vi "charsquential.vi"() -> ()   [LabVIEW 2012]
uses:
  <vilib>/addons/Modulation/Digital/General/MT Generate PSK System Parameters(M).vi
  <instrlib>/niUSRP/niUSRP Write Tx Data (CDB Cluster).vi
  <vilib>/addons/Modulation/niDMT.lvlib
panel:
  out "Enter control signal (1,2 or 3)\n1. Power\n2. Trade Off\n3. Bandwidth 2":string
  in  "Tx Parameters 3":T1={"Tx IQ Sampling\nRate [s/sec]"=500000.0, "Tx Frequency [Hz]"=2500000000.0, "Tx Gain [dB]"=0.0, "Tx Antenna"="TX1"} {"Tx Gain [dB]" format="%#.6p"; "Tx Frequency [Hz]" format="%#.6p"; "Tx IQ Sampling\nRate [s/sec]" format="%#.6p"}
  in  "Tx Parameters 2":T1={"Tx IQ Sampling\nRate [s/sec]"=500000.0, "Tx Frequency [Hz]"=2500000000.0, "Tx Gain [dB]"=0.0, "Tx Antenna"="TX1"} {"Tx Gain [dB]" format="%#.6p"; "Tx Frequency [Hz]" format="%#.6p"; "Tx IQ Sampling\nRate [s/sec]" format="%#.6p"}
  out "M-PSK (4)":i32
  out "Message Text 3":string="Two roads diverged in a yellow wood,\nAnd sorry I could not travel both\nAnd be one traveler, long I stood\nAnd looked down one as far as I could\nTo where it bent in the undergrowth.\n\nThen took the other, as just as fair,\nAnd having perhaps the better claim,\nBecause it was grassy and wanted wear;\nThough as for that the passing there\nHad worn them really about the same.\n\nAnd both that morning equally lay\nIn leaves no step had trodden black.\nOh, I kept the first for another day!\nYet knowing how way leads on to way,\nI doubted if I should ever come back.\n\nI shall be telling this with a sigh\nSomewhere ages and ages hence:\nTwo roads diverged in a wood, and I--\nI took the one less traveled by,\nAnd that has made all the difference.\n"
  out "x = y?":bool
  out "Boolean":bool
  out "millisecond timer value 2":u32
  in  "millisecond multiple 2":u32
  out "result":bool
  in  "BPSK System Parameters 9":T2={"Samples per Symbol"=8, "symbol map"=[], "Differential PSK"=enum."disable", "PSK type"=0} caption="BPSK System Parameters" {"PSK type" items=["normal", "shifted", "offset"]; "symbol map" format="%.3f"}
  in  "BPSK System Parameters 8":T2={"Samples per Symbol"=8, "symbol map"=[], "Differential PSK"=enum."disable", "PSK type"=0} caption="BPSK System Parameters" {"PSK type" items=["normal", "shifted", "offset"]; "symbol map" format="%.3f"}
  in  "BPSK System Parameters 7":T2={"Samples per Symbol"=8, "symbol map"=[], "Differential PSK"=enum."disable", "PSK type"=0} caption="BPSK System Parameters" {"PSK type" items=["normal", "shifted", "offset"]; "symbol map" format="%.3f"}
  in  "BPSK System Parameters 6":T2={"Samples per Symbol"=8, "symbol map"=[], "Differential PSK"=enum."disable", "PSK type"=0} caption="BPSK System Parameters" {"PSK type" items=["normal", "shifted", "offset"]; "symbol map" format="%.3f"}
  in  "BPSK System Parameters 5":T2={"Samples per Symbol"=8, "symbol map"=[], "Differential PSK"=enum."disable", "PSK type"=0} caption="BPSK System Parameters" {"PSK type" items=["normal", "shifted", "offset"]; "symbol map" format="%.3f"}
  in  "BPSK System Parameters 4":T2={"Samples per Symbol"=8, "symbol map"=[], "Differential PSK"=enum."disable", "PSK type"=0} caption="BPSK System Parameters" {"PSK type" items=["normal", "shifted", "offset"]; "symbol map" format="%.3f"}
  in  "BPSK System Parameters 3":T2={"Samples per Symbol"=8, "symbol map"=[], "Differential PSK"=enum."disable", "PSK type"=0} caption="BPSK System Parameters" {"PSK type" items=["normal", "shifted", "offset"]; "symbol map" format="%.3f"}
  out "String":string
  in  "millisecond multiple":u32
  out "millisecond timer value":u32
  in  "Tab Control":T3(tab)
  in  "Enter control signal (1,2 or 3)\n1. Power\n2. Trade Off\n3. Bandwidth":string
  in  "Packet Parameters":T4={"Guard Bits "=30, "Sync Bits"=20, "Message Bits"=128}
  in  "Packet Pad \n[samples]":i32=200
  in  "Blank Frame \n[samples]":i32=500
  out "Number of Packets in Message":i32=46
  in  "PN sequence order\nfor Sync Bits":i32=31 caption="PN sequence order (9)"
  in  "Packet Repeat":i32=2
  in  "Pulse Shaping Filter Parameters":T5={"Alpha"=0.5, "Filter Length"=6, "TX Filter"=enum."Root Raised Cos"} caption="Pulse Shaping Filter" {"Alpha" format="%.2f"}
  in  "Tx Parameters":T1={"Tx IQ Sampling\nRate [s/sec]"=500000.0, "Tx Frequency [Hz]"=2500000000.0, "Tx Gain [dB]"=0.0, "Tx Antenna"="TX1"} {"Tx Gain [dB]" format="%#.6p"; "Tx Frequency [Hz]" format="%#.6p"; "Tx IQ Sampling\nRate [s/sec]" format="%#.6p"}
  out "Actual Tx Parameters":T1={"Tx IQ Sampling\nRate [s/sec]"=200000.0, "Tx Frequency [Hz]"=2500000000.0, "Tx Gain [dB]"=0.0, "Tx Antenna"="TX1"} {"Tx Gain [dB]" format="%#.6p"; "Tx Frequency [Hz]" format="%#.6p"; "Tx IQ Sampling\nRate [s/sec]" format="%#.6p"}
  in  "USRP IP address":refnum<k15>="192.168.10.2"
  out "error out":errorcluster
  in  "Queue Length":i32=10
  out "Constellation Graph":T6(graph)
  in  "autoscale":bool
  out "Symbol Rate\n[symbols/sec]":dbl=25000.0 format="%#.6p"
  in  "stop":bool
  # "Guard\nBand"
  # "Sync\nSeq"
  # "Packet\nNumber"
  # "Pad\nData"
  # "Blank\nFrame"
  # "Data"
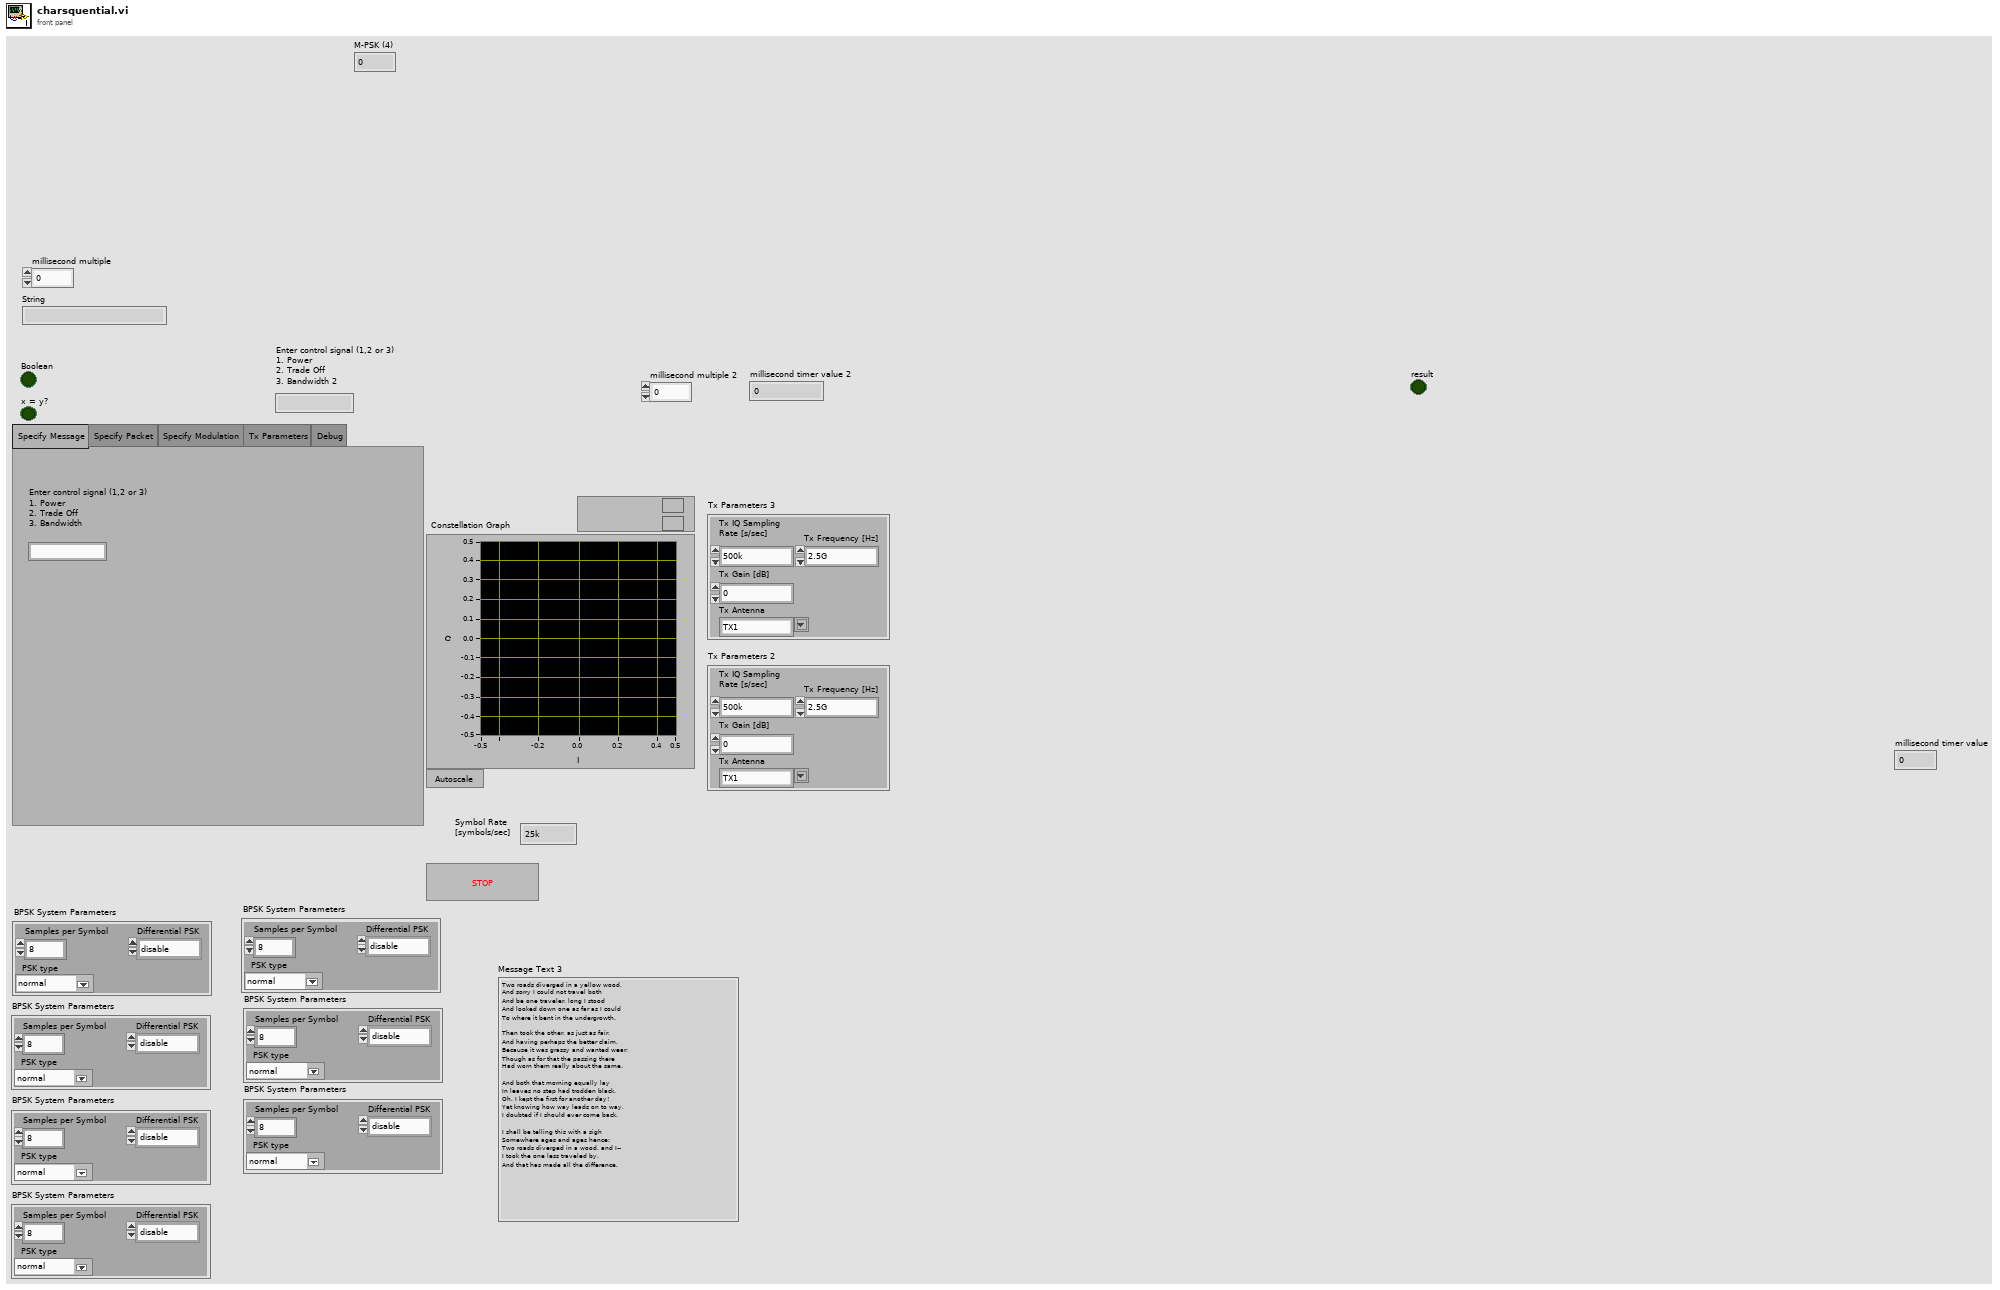
[diagram p1: front panel]
types:
  T1 = cluster{"Tx IQ Sampling\nRate [s/sec]":dbl, "Tx Frequency [Hz]":dbl, "Tx Gain [dB]":dbl, "Tx Antenna":string}
  T2 = cluster{"Samples per Symbol":i32, "symbol map":cdb[], "Differential PSK":enum16{"disable", "enable"}, "PSK type":u16}
  T3 = enum32{"Specify Message", "Specify Packet", "Specify Modulation", "Tx Parameters", "Debug"}
  T4 = cluster{"Guard Bits ":i32, "Sync Bits":i32, "Message Bits":i32}
  T5 = cluster{"Alpha":dbl, "Filter Length":i32, "TX Filter":enum16{"none", "Raised Cosine", "Root Raised Cos", "Gaussian"}}
  T6 = cluster{"Decimated Array":dbl[], "Decimated Array":dbl[]}[]
  T7 = cluster{"samples per symbol (16)":i32, "symbol map":cdb[], "differential PSK":enum16{"disable", "enable"}, "PSK type":u16}
  T8 = cluster{"s? t:f":cluster{"t0":dbl, "dt":dbl, "Y":cdb[]}, i32}
  T9 = cluster{"output complex waveform":cluster{"t0":dbl, "dt":dbl, "Y":cdb[]}, i32}
  T10 = cluster{"constellation":dbl[], "oversampled data":dbl[]}[]
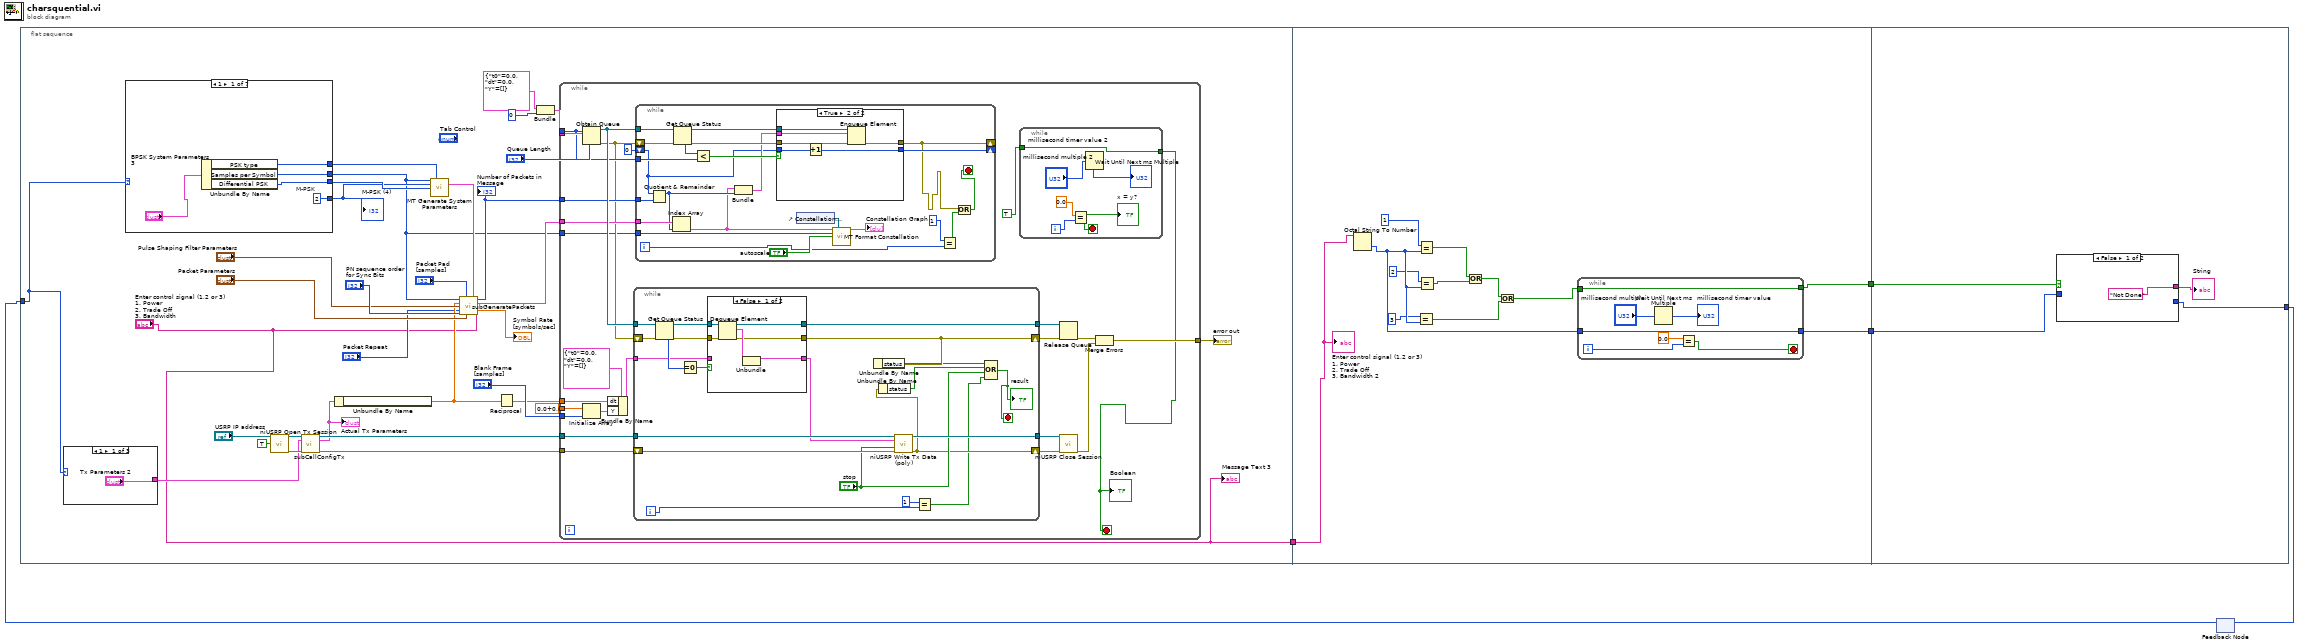
[diagram p0: block diagram]
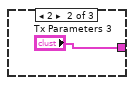
[diagram p2: hidden frame]
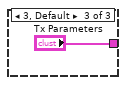
[diagram p3: hidden frame]
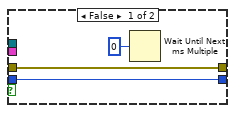
[diagram p4: hidden frame]
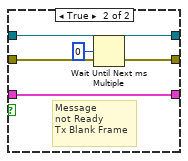
[diagram p5: hidden frame]
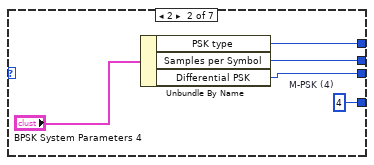
[diagram p6: hidden frame]
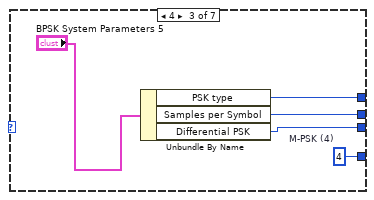
[diagram p7: hidden frame]
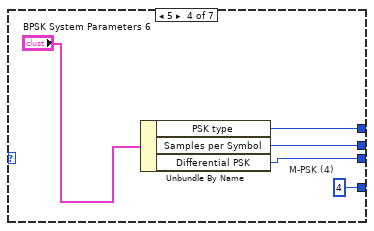
[diagram p8: hidden frame]
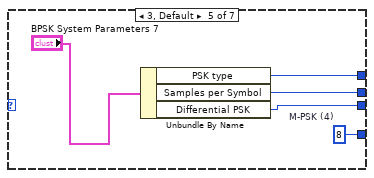
[diagram p9: hidden frame]
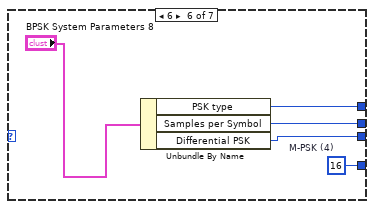
[diagram p10: hidden frame]
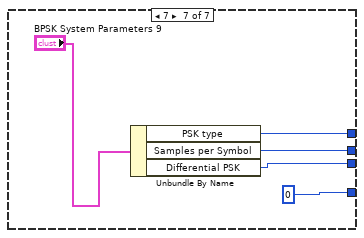
[diagram p11: hidden frame]
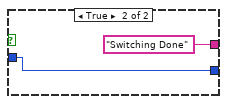
[diagram p12: hidden frame]
diagram:
  n1 = flat-sequence {
    tunnel: ["Enter control signal (1,2 or 3)\n1. Power\n2. Trade Off\n3. Bandwidth"] -> w5
    tunnel: w1 -> [w8]
    tunnel: w5 -> [w170]
    tunnel: [w172] -> w4
    tunnel: [w171] -> w3
    tunnel: w4 -> [w191]
    tunnel: w3 -> [w190]
    tunnel: [w189] -> w2
    frame #0 {
      n2 = case shown="1" w8 {
        tunnel: ["Tx Parameters 2" "Tx Parameters 3" "Tx Parameters"] -> w7
        frame 1 {
        }
        frame 2 {
        }
        frame 3, Default {
        }
      }
      n3 = case shown="1" w8 {
        tunnel: [w136 w141 w148 w153 w158 w164 w167] -> w11
        tunnel: [w137 w142 w147 w152 w157 w163 w168] -> w37
        tunnel: [w139 w144 w149 w154 w156 w162 0 ("M-PSK (4)")] -> w28
        tunnel: [w138 w143 w146 w151 w159 w161 w169] -> w17
        frame 1 {
          w139 = 2  # M-PSK
          n4 = Unbundle By Name("BPSK System Parameters 3") -> ("PSK type"=w138:u16, "Samples per Symbol"=w136:i32, "Differential PSK"=w137:enum16{"disable", "enable"})
        }
        frame 2 {
          w144 = 4  # M-PSK (4)
          n5 = Unbundle By Name("BPSK System Parameters 4") -> ("PSK type"=w143:u16, "Samples per Symbol"=w141:i32, "Differential PSK"=w142:enum16{"disable", "enable"})
        }
        frame 4 {
          w149 = 4  # M-PSK (4)
          n6 = Unbundle By Name("BPSK System Parameters 5") -> ("PSK type"=w146:u16, "Samples per Symbol"=w148:i32, "Differential PSK"=w147:enum16{"disable", "enable"})
        }
        frame 5 {
          w154 = 4  # M-PSK (4)
          n7 = Unbundle By Name("BPSK System Parameters 6") -> ("PSK type"=w151:u16, "Samples per Symbol"=w153:i32, "Differential PSK"=w152:enum16{"disable", "enable"})
        }
        frame 3, Default {
          w156 = 8  # M-PSK (4)
          n8 = Unbundle By Name("BPSK System Parameters 7") -> ("PSK type"=w159:u16, "Samples per Symbol"=w158:i32, "Differential PSK"=w157:enum16{"disable", "enable"})
        }
        frame 6 {
          w162 = 16  # M-PSK (4)
          n9 = Unbundle By Name("BPSK System Parameters 8") -> ("PSK type"=w161:u16, "Samples per Symbol"=w164:i32, "Differential PSK"=w163:enum16{"disable", "enable"})
        }
        frame 7 {
          n10 = Unbundle By Name("BPSK System Parameters 9") -> ("PSK type"=w169:u16, "Samples per Symbol"=w167:i32, "Differential PSK"=w168:enum16{"disable", "enable"})
        }
      }
      "M-PSK (4)" <- w28
      n11 = call <instrlib>:"niUSRP Open Tx Session.vi"("device names"="USRP IP address", "reset"=TRUE) -> ("session handle out"=w21:refnum<k15>, "error out"=w20:errorcluster)  [unwired: 12 in]
      n12 = call "subCallConfigTx.vi"("session handle"=w21, "Tx Parameters"=w7, "error in"=w20) -> ("session handle out"=w27:refnum<k15>, "Actual Tx Parameters"=w26:T1, "error out"=w30:errorcluster)  [unwired: 10 in]
      "Actual Tx Parameters" <- w26
      n13 = Unbundle By Name(w26) -> ("Tx IQ Sampling\nRate [s/sec]"=w12:dbl)
      n14 = call-poly <vilib>:"MT Generate System Parameters.vi"("samples per symbol (16)"=w11, "PSK type"=w17, "M-PSK (4)"=w28, "differential PSK"=w37) -> ("PSK system parameters"=w18:T7)  [unwired: 9 in, 2 out]
      n15 = call "subGeneratePackets.vi"("Samples per Symbol"=w11, "Packet Pad \n[samples]"="Packet Pad \n[samples]", "PSK system parameters"=w18, "Tx IQ Sampling\nRate [s/sec]"=w12, "Pulse Shaping Filter Parameters"="Pulse Shaping Filter Parameters", "Packet Repeat"="Packet Repeat", "PN sequence order\nfor Sync Bits"="PN sequence order\nfor Sync Bits", "Packet Parameters"="Packet Parameters", "Message Text"="Enter control signal (1,2 or 3)\n1. Power\n2. Trade Off\n3. Bandwidth") -> ("Number of Packets"=w25:i32, "Packets"=w31:cluster{"t0":dbl, "dt":dbl, "Y":cdb[]}[], "Symbol Rate"=→"Symbol Rate\n[symbols/sec]":dbl)  [unwired: 4 in]
      "Number of Packets in Message" <- w25
      n16 = Reciprocal(x=w12) -> (1/x=w29:dbl)
      n17 = Bundle("s? t:f"=cluster{"t0":dbl, "dt":dbl, "Y":cdb[]} {"t0"=0.0, "dt"=0.0, "Y"=[]}, 0) -> (w33:T8)  [unwired: 1 in]
      n18 = while {
        tunnel: cdb 0.0+0.0i ("element") -> [w65]
        tunnel: "Blank Frame \n[samples]" -> [w64]
        tunnel: w33 -> [w58]
        tunnel: "Queue Length" -> [w56]
        tunnel: w31 -> [w55]
        tunnel: w30 -> [w54]
        tunnel: w29 -> [w51]
        tunnel: w27 -> [w50]
        tunnel: w25 -> [w49]
        tunnel: [w44] -> w16
        tunnel: w11 -> [w43]
        stop <- w41 stop-if-true
        n19 = Obtain Queue(max queue size (-1, unlimited)=w56, element data type=w58) -> (queue out=w63:refnum<queue>, error out=w47:errorcluster)  [unwired: 3 in, 1 out]
        n20 = Initialize Array(w65, w64) -> (w62:cdb[])
        n21 = Bundle By Name(cluster=cluster{"t0":dbl, "dt":dbl, "Y":cdb[]} {"t0"=0.0, "dt"=0.0, "Y"=[]} ("s? t:f"), "dt"=w51, "Y"=w62) -> (w61:cluster{"t0":dbl, "dt":dbl, "Y":cdb[]})
        n22 = while {
          tunnel: w50 -> [w115]
          shift-right: [w106] -> w53
          shift-left: w54 -> [w116]
          tunnel: w63 -> [w124]
          tunnel: w61 -> [w121]
          tunnel: [w120] -> w60
          tunnel: [w114] -> w52
          shift-right: [w111] -> w59
          shift-left: w47 -> [w117]
          i -> [w108]
          stop <- w104 stop-if-true
          n23 = Get Queue Status(queue=w124, error in (no error)=w117) -> (queue out=w119:refnum<queue>, error out=w118:errorcluster, # elements in queue=w123:i32)  [unwired: 1 in, 5 out]
          n24 = Equal To 0?(x=w123) -> (x = 0?=w122:bool)
          n25 = case shown="False" w122 {
            tunnel: w121 -> [_ w134]
            tunnel: [w126 w134] -> w109
            tunnel: [w130 w132] -> w120
            tunnel: [w125 w133] -> w111
            tunnel: w119 -> [w129 w132]
            tunnel: w118 -> [w128 w133]
            frame False {
              n26 = Dequeue Element(queue=w129, error in (no error)=w128) -> (queue out=w130:refnum<queue>, element=w127:T8, error out=w125:errorcluster)  [unwired: 1 in, 1 out]
              n27 = Unbundle(w127) -> ("s? t:f"=w126:cluster{"t0":dbl, "dt":dbl, "Y":cdb[]})  [unwired: 1 out]
            }
            frame True {
              # "Message\nnot Ready\nTx Blank Frame"
              n28 = Wait Until Next ms Multiple(millisecond multiple=u32 0) -> ()  [unwired: 1 out]
            }
          }
          n29 = Unbundle By Name(w111) -> ("status"=w110:bool)
          n30 = call-poly <instrlib>:"niUSRP Write Tx Data (poly).vi"("session handle"=w115, "data"=w109, "end of data?"="stop", "error in (no error)"=w116) -> ("session handle out"=w114:refnum<k15>, "error out"=w106:errorcluster)  [unwired: 10 in]
          n31 = Unbundle By Name(w106) -> ("status"=w113:bool)
          n32 = Equal?(x=1, y=w108) -> (x = y?=w105:bool)
          n33 = Compound Arithmetic op=OR(w110, w113, "stop", w105) -> (w104:bool)
          "result" <- w104
        }
        n34 = while {
          tunnel: w63 -> [w94]
          shift-right: [w87] -> _
          shift-left: 0 -> [w83]
          tunnel: w55 -> [w84]
          tunnel: w56 -> [w86]
          tunnel: w49 -> [w85]
          shift-right: [w75] -> _
          shift-left: w47 -> [w89]
          tunnel: w43 -> [w79]
          i -> [w72]
          stop <- w74 stop-if-true
          n35 = Quotient & Remainder(x=w83, y=w85) -> (x-y*floor(x/y)=w82:i32)  [unwired: 1 out]
          n36 = Index Array(array=w84, index=w82) -> (element=w77:cluster{"t0":dbl, "dt":dbl, "Y":cdb[]})
          n37 = Get Queue Status(queue=w94, error in (no error)=w89) -> (queue out=w93:refnum<queue>, error out=w90:errorcluster, # elements in queue=w92:i32)  [unwired: 1 in, 5 out]
          n38 = Less?(x=w92, y=w86) -> (x < y?=w91:bool)
          n39 = Bundle("output complex waveform"=w77, w82) -> (w88:T9)  [unwired: 1 in]
          n40 = case shown="True" w91 {
            tunnel: w90 -> [w95 w103]
            tunnel: w93 -> [_ w102]
            tunnel: [w95 w101] -> w75
            tunnel: w88 -> [_ w100]
            tunnel: w83 -> [w97 w99]
            tunnel: [w97 w98] -> w87
            frame False {
              n41 = Wait Until Next ms Multiple(millisecond multiple=u32 0) -> ()  [unwired: 1 out]
            }
            frame True {
              n42 = Increment(x=w99) -> (x+1=w98:i32)
              n43 = Enqueue Element(queue=w102, element=w100, error in (no error)=w103) -> (error out=w101:errorcluster)  [unwired: 1 in, 2 out]
            }
          }
          n44 = control-ref of="Constellation Graph"() -> (w80:refnum<vi>)
          n45 = call <vilib>:"MT Format Constellation.vi"("waveform"=w77, "constellation reference"=w80, "samples per symbol"=w79, "autoscale"="autoscale") -> ("constellation graph"=→"Constellation Graph":T10)  [unwired: 1 in, 10 out]
          n46 = Equal?(x=1, y=w72) -> (x = y?=w76:bool)
          n47 = Or(x=w75, y=w76) -> (x .or. y?=w74:bool)
        }
        n48 = while {
          tunnel: TRUE -> [w71]
          tunnel: [w71] -> w41
          i -> [w69]
          stop <- w68 stop-if-true
          n49 = Equal?(x=0.0, y=w69) -> (x = y?=w68:bool)
          "x = y?" <- w68
          n50 = Wait Until Next ms Multiple(millisecond multiple="millisecond multiple 2") -> (millisecond timer value=→"millisecond timer value 2":u32)
        }
        "Boolean" <- w41
        n51 = Release Queue(queue=w60, error in (no error)=w59) -> (error out=w46:errorcluster)  [unwired: 3 out]
        n52 = call <instrlib>:"niUSRP Close Session.vi"("session handle"=w52, "error in (no error)"=w53) -> ("error out"=w45:errorcluster)  [unwired: 13 in]
        n53 = Merge Errors(w46, w45) -> (w44:errorcluster)
      }
      "error out" <- w16
      "Message Text 3" <- "Enter control signal (1,2 or 3)\n1. Power\n2. Trade Off\n3. Bandwidth"
    }
    frame #1 {
      n54 = Octal String To Number(4:w170) -> (0:w176:u32)  [unwired: 2 in, 1 out]
      n55 = Equal?(x=3, y=w176) -> (x = y?=w178:bool)
      n56 = Equal?(x=1, y=w176) -> (x = y?=w181:bool)
      n57 = Equal?(x=2, y=w176) -> (x = y?=w180:bool)
      n58 = Or(x=w181, y=w180) -> (x .or. y?=w179:bool)
      n59 = Or(x=w179, y=w178) -> (x .or. y?=w177:bool)
      n60 = while {
        tunnel: w177 -> [w186]
        tunnel: [w186] -> w172
        tunnel: w176 -> [w185]
        tunnel: [w185] -> w171
        i -> [w183]
        stop <- w182 stop-if-true
        n61 = Wait Until Next ms Multiple(millisecond multiple="millisecond multiple") -> (millisecond timer value=→"millisecond timer value":u32)
        n62 = Equal?(x=0.0, y=w183) -> (x = y?=w182:bool)
      }
      "Enter control signal (1,2 or 3)\n1. Power\n2. Trade Off\n3. Bandwidth 2" <- w170
    }
    frame #2 {
      n63 = case shown="False" w191 {
        tunnel: ["Not Done" "Switching Done"] -> w192
        tunnel: [_ w194] -> w189
        tunnel: w190 -> [_ w194]
        frame False {
        }
        frame True {
        }
      }
      "String" <- w192
    }
  }
  n64 = feedback-in #1(w2) -> ()
  n65 = feedback #1() -> (w1:u32)  [unwired: 1 in]
